vi "hydrolyse_reactor_setup.vi"(10 "#":i32) -> (2 "spec_file":path)   [LabVIEW 2019]
uses:
  lib/libSimulationControl/libSimulationControl.lvlib
  lib/libCheckpointUpdate/libCheckpointUpdate.lvlib
panel:
  # "*******************************************************************\nBiogas Plant Control\n\nAuthor: Paul Zügel\nGCSC-Frankfurt am Main 2020\n\n*******************************************************************"
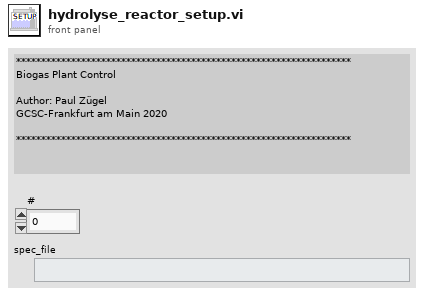
[diagram p1: front panel]
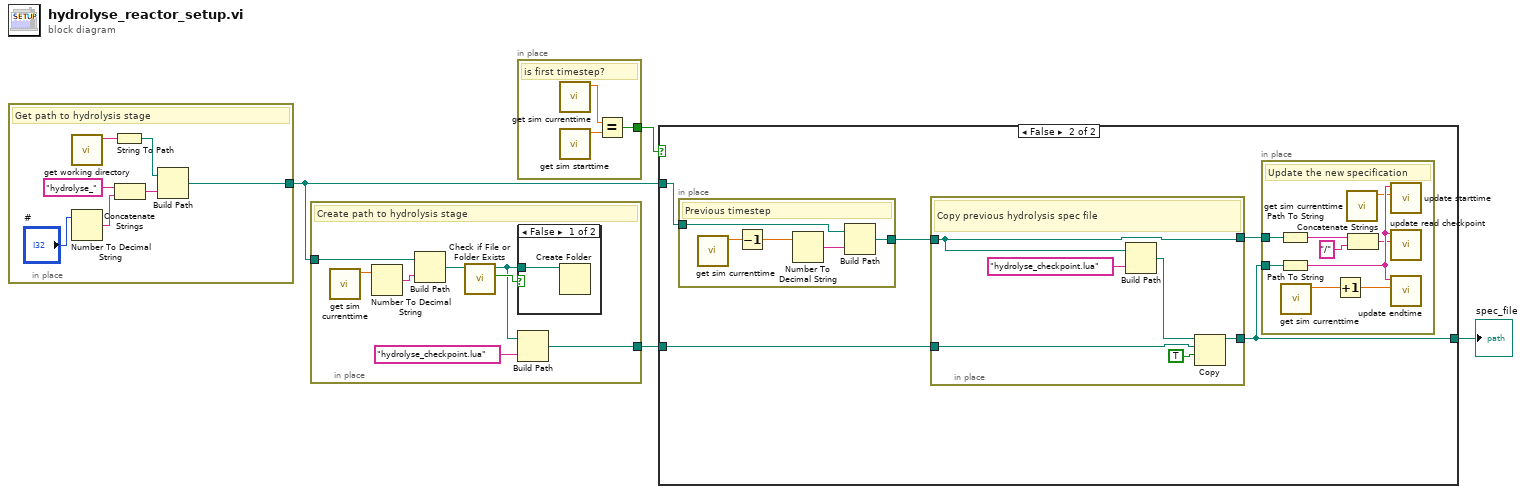
[diagram p0: block diagram]
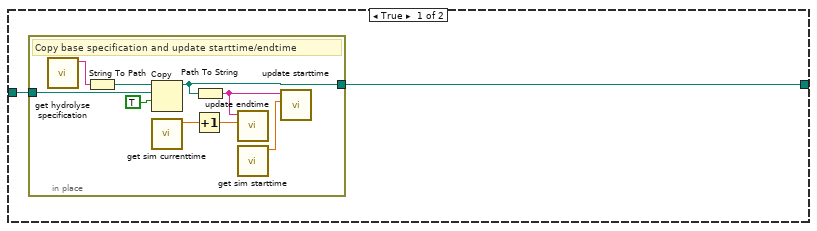
[diagram p3: hidden frame]
diagram:
  n1 = in-place {
    in-place-border: [w5] -> w1
    # "Get path to hydrolysis stage"
    n2 = call "get working directory.vi"() -> ("function return"=w10:string)  [unwired: 10 in, 1 out]
    n3 = Number To Decimal String(number="#") -> (decimal integer string=w11:string)  [unwired: 1 in]
    n4 = String To Path(string=w10) -> (path=w6:path)
    n5 = Concatenate Strings("hydrolyse_" ("string"), w11) -> (w9:string)
    n6 = Build Path(base path=w6, name or relative path=w9) -> (appended path=w5:path)
  }
  n7 = in-place {
    in-place-border: [w14] -> w3
    in-place-border: w1 -> [w12]
    # "Create path to hydrolysis stage"
    n8 = call "get sim currenttime.vi"() -> ("current_time"=w13:dbl)  [unwired: 10 in, 1 out]
    n9 = Number To Decimal String(number=w13) -> (decimal integer string=w18:string)  [unwired: 1 in]
    n10 = Build Path(base path=w12, name or relative path=w18) -> (appended path=w17:path)
    n11 = call <vilib>:"Check if File or Folder Exists.vi"("path"=w17) -> ("file or folder exists?"=w19:bool, "dup path"=w16:path)  [unwired: 8 in, 1 out]
    n12 = case shown="False" w19 {
      tunnel: w16 -> [w20 _]
      frame False {
        n13 = Create Folder(path (use dialog)=w20) -> ()  [unwired: 2 in, 3 out]
      }
      frame True {
      }
    }
    n14 = Build Path(base path=w16, name or relative path="hydrolyse_checkpoint.lua" ("string")) -> (appended path=w14:path)
  }
  n15 = in-place {
    in-place-border: [w23] -> w4
    # "is first timestep?"
    n16 = call "get sim currenttime.vi"() -> ("current_time"=w21:dbl)  [unwired: 10 in, 1 out]
    n17 = call "get sim starttime.vi"() -> ("sim_starttime"=w22:dbl)  [unwired: 10 in, 1 out]
    n18 = Equal?(x=w21, y=w22) -> (x = y?=w23:bool)
  }
  n19 = case shown="False" w4 {
    tunnel: w3 -> [w25 w37]
    tunnel: [w24 w36] -> w2
    tunnel: w1 -> [_ w35]
    frame True {
      n20 = in-place {
        in-place-border: [w33] -> w24
        in-place-border: w25 -> [w26]
        # "Copy base specification and update starttime/endtime"
        n21 = call "get hydrolyse specification.vi"() -> ("function return"=w27:string)  [unwired: 10 in, 1 out]
        n22 = String To Path(string=w27) -> (path=w34:path)
        n23 = Copy(9:TRUE ("overwrite (F)"), 10:w26, 11:w34) -> (3:w33:path)  [unwired: 2 in, 2 out]
        n24 = call "get sim currenttime.vi"() -> ("current_time"=w29:dbl)  [unwired: 10 in, 1 out]
        n25 = Increment(x=w29) -> (x+1=w28:dbl)
        n26 = Path To String(path=w33) -> (string=w30:string)
        n27 = call "update endtime.vi"("endtime"=w28, "spec_dir"=w30) -> ()  [unwired: 9 in, 1 out]
        n28 = call "get sim starttime.vi"() -> ("sim_starttime"=w31:dbl)  [unwired: 10 in, 1 out]
        n29 = call "update starttime.vi"("starttime"=w31, "spec_dir"=w30) -> ()  [unwired: 9 in, 1 out]
      }
    }
    frame False {
      n30 = in-place {
        in-place-border: [w51] -> w39
        in-place-border: w35 -> [w49]
        # "Previous timestep"
        n31 = call "get sim currenttime.vi"() -> ("current_time"=w50:dbl)  [unwired: 10 in, 1 out]
        n32 = Decrement(x=w50) -> (x-1=w53:dbl)
        n33 = Number To Decimal String(number=w53) -> (decimal integer string=w52:string)  [unwired: 1 in]
        n34 = Build Path(base path=w49, name or relative path=w52) -> (appended path=w51:path)
      }
      n35 = in-place {
        in-place-border: w39 -> [w57]
        in-place-border: [w57] -> w38
        in-place-border: w37 -> [w55]
        in-place-border: [w54] -> w36
        # "Copy previous hydrolysis spec file"
        n36 = Build Path(base path=w57, name or relative path="hydrolyse_checkpoint.lua" ("string")) -> (appended path=w58:path)
        n37 = Copy(9:TRUE ("overwrite (F)"), 10:w55, 11:w58) -> (3:w54:path)  [unwired: 2 in, 2 out]
      }
      n38 = in-place {
        in-place-border: w38 -> [w47]
        in-place-border: w36 -> [w40]
        # "Update the new specification"
        n39 = Path To String(path=w47) -> (string=w46:string)
        n40 = Path To String(path=w40) -> (string=w48:string)
        n41 = call "get sim currenttime.vi"() -> ("current_time"=w42:dbl)  [unwired: 10 in, 1 out]
        n42 = Increment(x=w42) -> (x+1=w41:dbl)
        n43 = call "get sim currenttime.vi"() -> ("current_time"=w43:dbl)  [unwired: 10 in, 1 out]
        n44 = Concatenate Strings(w46, "/" ("string")) -> (w44:string)
        n45 = call "update starttime.vi"("starttime"=w43, "spec_dir"=w48) -> ()  [unwired: 9 in, 1 out]
        n46 = call "update read checkpoint.vi"("checkpoint_dir"=w44, "spec_dir"=w48) -> ()  [unwired: 9 in, 1 out]
        n47 = call "update endtime.vi"("endtime"=w41, "spec_dir"=w48) -> ()  [unwired: 9 in, 1 out]
      }
    }
  }
  "spec_file" <- w2
